vi "String to Tree.VI"(2 "error in (no error)":errorcluster, 3 "user formula":string) -> (0 "error out":errorcluster, 1 "Tree formula":T1(array[cluster]))   [LabVIEW 2014, in "NI_Gmath.lvlib"]
uses:
  NI_Gmath.lvlib
panel:
  out "error in formula":string
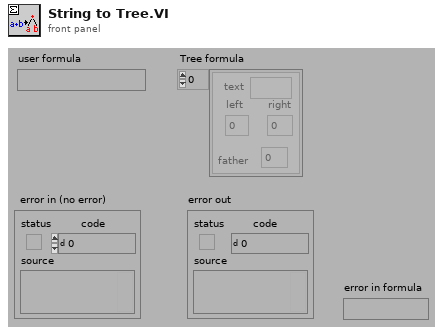
[diagram p1: front panel]
types:
  T1 = cluster{"text":string, "left":i32, "right":i32, "father":i32}[]
  T2 = cluster{"text":string, "left":i32, "right":i32, "father":i32}
  T3 = cluster{bool, i32, "error in formula-write":string}
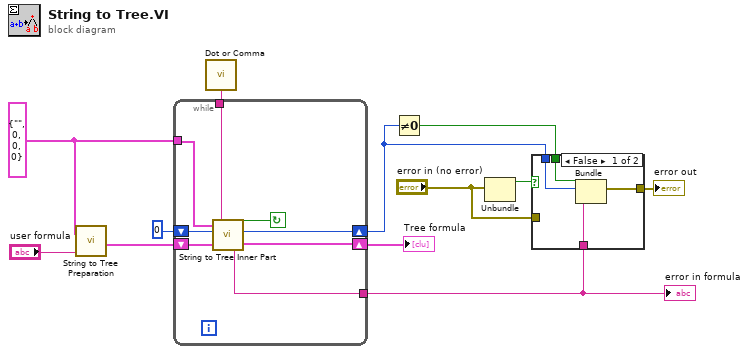
[diagram p0: block diagram]
diagram:
  w2 = T2 {"text"="", "left"=0, "right"=0, "father"=0} ("dummy")
  n1 = call "String to Tree Preparation.vi"("user formula"="user formula", "dummy"=w2) -> ("empty structure"=w12:T1)
  n2 = call "Dot or Comma.vi"() -> ("dot or comma"=w4:string)
  n3 = while {
    tunnel: w4 -> [w15]
    shift-left: 0 -> [w17]
    shift-right: [w18] -> w6
    tunnel: w2 -> [w20]
    shift-left: w12 -> [w19]
    shift-right: [w14] -> w3
    tunnel: [w13] -> w1
    stop <- w16 continue-if-true
    n4 = call "String to Tree Inner Part.vi"("structure before"=w19, "dummy"=w20, "error situation before"=w17, "dot or comma"=w15) -> ("error in formula-write"=w13:string, "structure after"=w14:T1, "error situation after"=w18:i32, "end of analysis"=w16:bool)
  }
  "Tree formula" <- w3
  "error in formula" <- w1
  n5 = Not Equal To 0?(x=w6) -> (x != 0?=w5:bool)
  n6 = Unbundle("error in (no error)") -> ("status"=w9:bool)  [unwired: 2 out]
  n7 = case shown="False" w9 {
    tunnel: "error in (no error)" -> [_ w25]
    tunnel: [w24 w25] -> w7
    tunnel: w6 -> [w23 _]
    tunnel: w5 -> [w22 _]
    tunnel: w1 -> [w21 _]
    frame False {
      n8 = Bundle(w22, w23, "error in formula-write"=w21) -> (w24:T3)  [unwired: 1 in]
    }
    frame True {
    }
  }
  "error out" <- w7
